vi "Toggle.vi"(8 "error in (no error)":errorcluster, 10 "Dirrection":enum16{"Forward", "Reverse"}(ring), 11 "State in":refnum<class "Child Actor.lvclass">) -> (0 "error out":errorcluster, 3 "State out":refnum<class "Child Actor.lvclass">)   [LabVIEW 2015, in "Child Actor.lvclass"]
uses:
  Child Actor.lvclass
  State/Parent Actor.lvclass
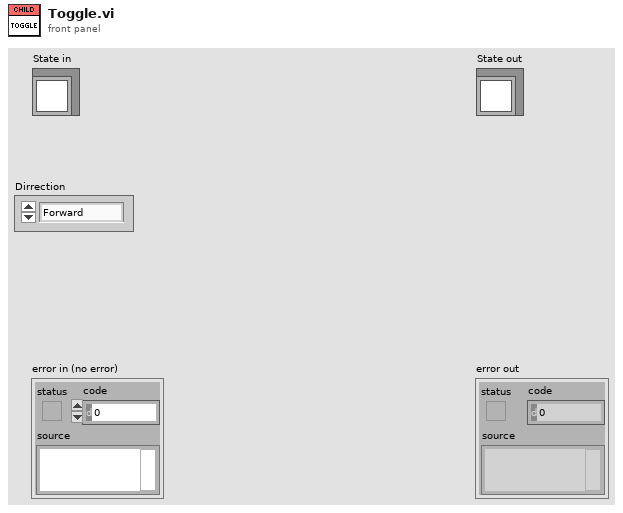
[diagram p1: front panel]
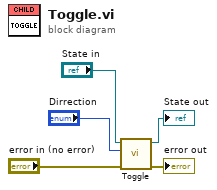
[diagram p0: block diagram]
diagram:
  n1 = call-parent "Toggle.vi"("error in (no error)"="error in (no error)", "Dirrection"="Dirrection", "State in"="State in") -> ("error out"=→"error out":errorcluster, "State out"=→"State out":refnum<class "Child Actor.lvclass">)  [unwired: 7 in]
